vi "Rotation Matrix to Fick.vi"(5 "A":dbl[][](array[numeric]) format="%.2f") -> (0 "T":dbl format="%.2f", 1 "V":dbl format="%.2f", 2 "H":dbl format="%.2f")   [LabVIEW 2013, in "fick-matrix.lvlib"]
uses:
  fick-matrix.lvlib
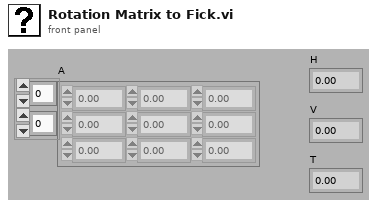
[diagram p1: front panel]
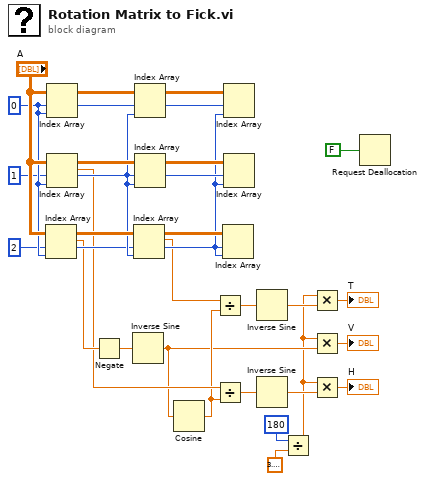
[diagram p0: block diagram]
diagram:
  w18 = 2
  w19 = 1
  w20 = 0
  n1 = Index Array(array="A", index (row)=w18, index (col)=w20) -> (element=w17:dbl)
  n2 = Index Array(array="A", index (row)=w20, index (col)=w20) -> ()  [unwired: 1 out]
  n3 = Index Array(array="A", index (row)=w19, index (col)=w20) -> (element=w15:dbl)
  n4 = Negate(x=w17) -> (-x=w16:dbl)
  n5 = Inverse Sine(1:w16) -> (0:w7:dbl)
  n6 = Index Array(array="A", index (row)=w18, index (col)=w19) -> (element=w11:dbl)
  n7 = Index Array(array="A", index (row)=w20, index (col)=w19) -> ()  [unwired: 1 out]
  n8 = Index Array(array="A", index (row)=w19, index (col)=w19) -> ()  [unwired: 1 out]
  n9 = Cosine(x=w7) -> (cos(x)=w12:dbl)
  n10 = Divide(x=w11, y=w12) -> (x/y=w13:dbl)
  n11 = Divide(x=w15, y=w12) -> (x/y=w14:dbl)
  n12 = Index Array(array="A", index (row)=w18, index (col)=w18) -> ()  [unwired: 1 out]
  n13 = Index Array(array="A", index (row)=w20, index (col)=w18) -> ()  [unwired: 1 out]
  n14 = Index Array(array="A", index (row)=w19, index (col)=w18) -> ()  [unwired: 1 out]
  n15 = Inverse Sine(1:w13) -> (0:w8:dbl)
  n16 = Inverse Sine(1:w14) -> (0:w6:dbl)
  n17 = Divide(x=180, y=3.141592653589793) -> (x/y=w5:dbl)
  n18 = Multiply(x=w5, y=w8) -> (x*y=→"T":dbl)
  n19 = Multiply(x=w5, y=w7) -> (x*y=→"V":dbl)
  n20 = Multiply(x=w5, y=w6) -> (x*y=→"H":dbl)
  n21 = Request Deallocation(FALSE ("flag")) -> ()
